vi "Create CLI Report.vi"(8 "error in (no error)":errorcluster, 10 "Results":T1[](array[typedef]) {"Time End" format="%<%x %.3X>T"; "Time Start" format="%<%x %.3X>T"}, 11 "Report Folder":path) -> (0 "error dub":errorcluster)   [LabVIEW 2020, in "ProjectBuilder.lvlib"]
uses:
  ProjectBuilder.lvlib
  Ctl/Ctl_Action Result.ctl
  Class/Action/Project Action/Project Action.lvclass
  Ctl/Ctl_Build Steps.ctl
  Class/Data/Report Data/Report Data.lvclass
  <vilib>/Utility/file.llb/Write Delimited Spreadsheet (string).vi
  PPL/HDH.ClassLoader.lvlibp
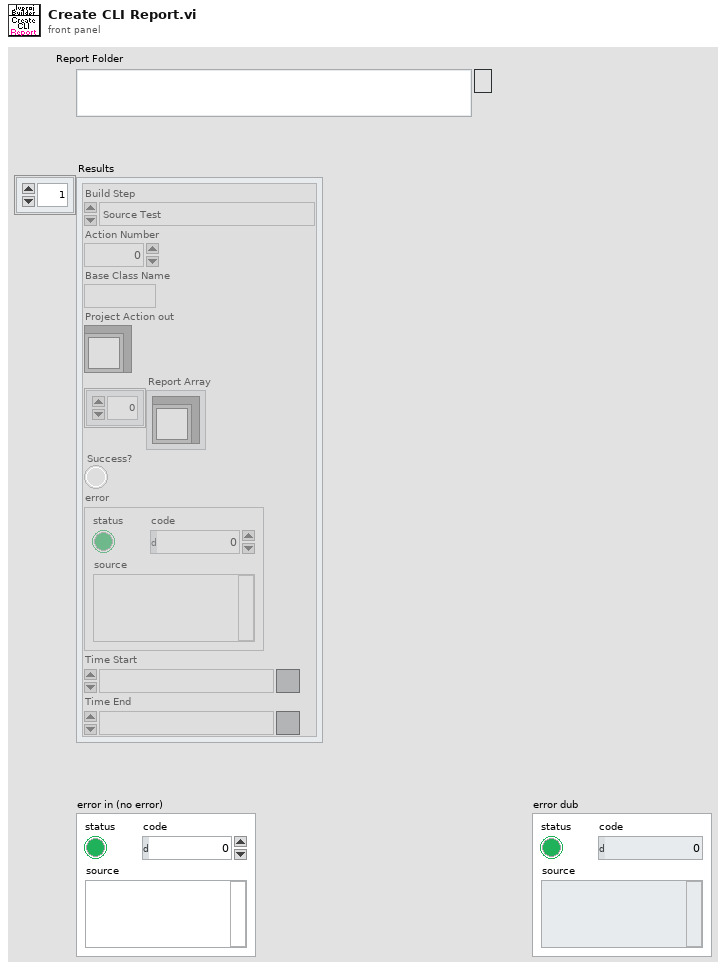
[diagram p1: front panel]
types:
  T1 = typedef "ProjectBuilder.lvlib/Ctl_Action Result.ctl" = cluster{"Build Step":T2, "Action Number":i32, "Base Class Name":string, "Project Action out":refnum<class "Project Action.lvclass">, "Report Array":refnum<class "Report Data.lvclass">[], "Success?":bool, "error":errorcluster, "Time Start":timestamp, "Time End":timestamp}
  T2 = typedef "ProjectBuilder.lvlib/Ctl_Build Steps.ctl" = enum16{"Source Test", "Build", "Post-Build Test", "Deploy", "Report"}
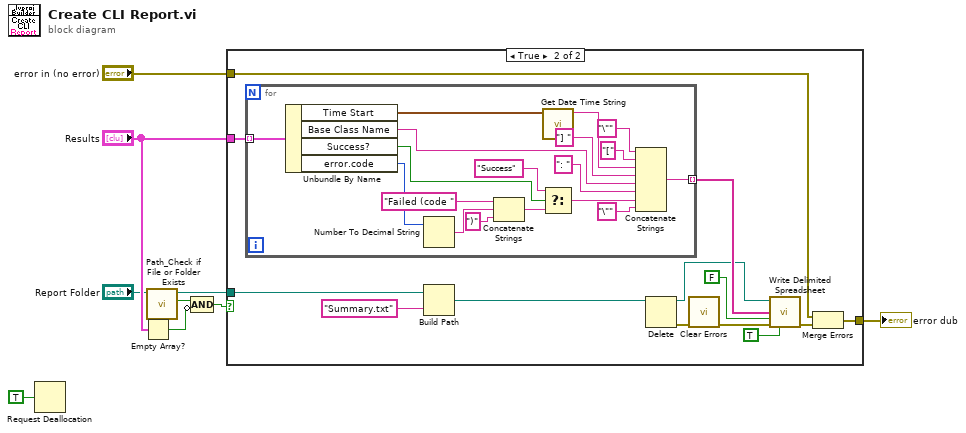
[diagram p0: block diagram]
diagram:
  n1 = Request Deallocation(TRUE ("flag")) -> ()
  n2 = Empty Array?(array="Results") -> (empty?=w8:bool)
  n3 = call "Path_Check if File or Folder Exists.vi"("File or Folder Path in"="Report Folder") -> ("File or Folder Found?"=w5:bool, "File or Folder Path dub"=w4:path)  [unwired: 9 in]
  n4 = Compound Arithmetic op=AND(w5, invert w8) -> (w7:bool)
  n5 = case shown="True" w7 {
    tunnel: "Results" -> [_ w23]
    tunnel: w4 -> [_ w21]
    tunnel: [w10 w17] -> w2
    tunnel: "error in (no error)" -> [w10 w18]
    frame False {
    }
    frame True {
      n6 = for {
        tunnel: w23 -> [w41] mode=indexing
        tunnel: [w26] -> w19 mode=indexing
        n7 = Unbundle By Name(w41) -> ("Time Start"=w40:timestamp, "Base Class Name"=w36:string, "Success?"=w34:bool, "error.code"=w32:i32)
        n8 = Number To Decimal String(number=w32) -> (decimal integer string=w30:string)  [unwired: 1 in]
        n9 = Concatenate Strings("Failed (code ", w30, ")" ("string")) -> (w28:string)
        n10 = call "Get Date Time String.vi"("Time (Current time)"=w40) -> ("Time String"=w38:string)  [unwired: 10 in]
        n11 = Select(t="Success", s=w34, f=w28) -> (s? t:f=w27:string)
        n12 = Concatenate Strings("\"" ("string"), "[" ("string"), w38, "] " ("string"), w36, ": " ("string"), w27, "\"" ("string")) -> (w26:string)
      }
      n13 = Build Path(base path=w21, name or relative path="Summary.txt") -> (appended path=w14:path)
      n14 = Delete(path (use dialog)=w14) -> (deleted path=w13:path, error out=w12:errorcluster)  [unwired: 4 in, 1 out]
      n15 = call <vilib>:"Clear Errors.vi"("error in (no error)"=w12) -> ("error out"=w11:errorcluster)  [unwired: 5 in, 1 out]
      n16 = call-poly <vilib>:"Write Delimited Spreadsheet.vi"("file path (dialog if empty)"=w13, "1D data"=w19, "append to file? (new file:F)"=FALSE, "error in (no error)"=w11, "transpose? (no:F)"=TRUE) -> ("error out"=w16:errorcluster)  [unwired: 9 in, 1 out]
      n17 = Merge Errors(w18, w16) -> (w17:errorcluster)
    }
  }
  "error dub" <- w2
